vi "ex14-3.vi"() -> ()   [LabVIEW 2014]
panel:
  out "二進位":dbl[](array[numeric])
  in  "十進位":dbl
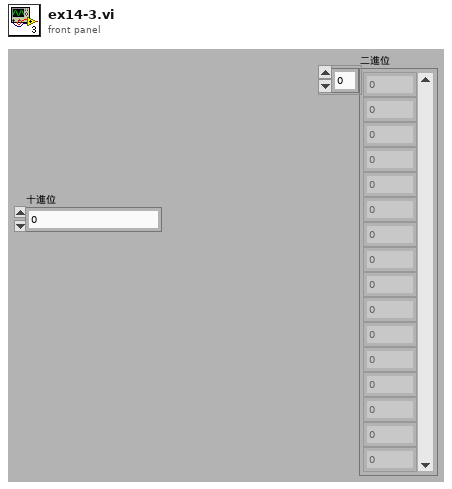
[diagram p1: front panel]
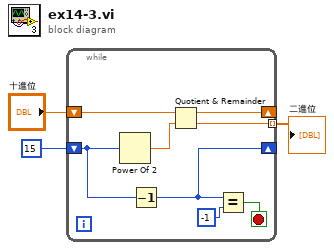
[diagram p0: block diagram]
diagram:
  n1 = while {
    shift-right: [w4] -> _
    shift-left: 15 -> [w11]
    shift-right: [w9] -> _
    shift-left: "十進位" -> [w8]
    tunnel: [w5] -> w1 mode=indexing
    stop <- w7 stop-if-true
    n2 = Power Of 2(x=w11) -> (2^x=w10:dbl)
    n3 = Decrement(x=w11) -> (x-1=w4:i32)
    n4 = Quotient & Remainder(x=w8, y=w10) -> (x-y*floor(x/y)=w9:dbl, floor(x/y)=w5:dbl)
    n5 = Equal?(x=w4, y=-1) -> (x = y?=w7:bool)
  }
  "二進位" <- w1
